vi "Read Base Name.vi"(8 "error in (no error)":errorcluster, 11 "Base In":refnum<class "Base.lvclass">) -> (0 "error out":errorcluster, 2 "Name":string, 3 "Base Out":refnum<class "Base.lvclass">)   [LabVIEW 2020, in "Base.lvclass"]
doc: "Returns the name of the object. The Qualified Name is prepended with the name of the owner recursively in the format \"Owner Name::Name\"."
uses:
  Base.lvclass
  Base.lvclass/Base.ctl
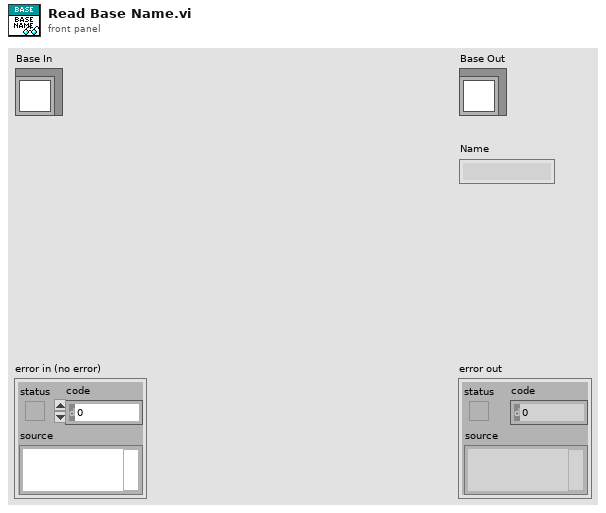
[diagram p1: front panel]
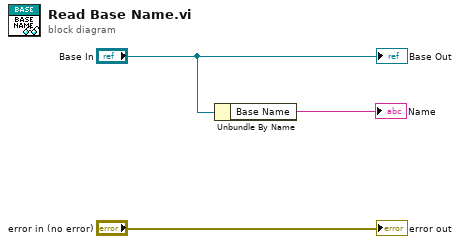
[diagram p0: block diagram]
diagram:
  n1 = Unbundle By Name("Base In") -> ("Base Name"=→"Name":string)
  "error out" <- "error in (no error)"
  "Base Out" <- "Base In"
